vi "PNA-L_SET-CWFREQ.vi"(0 "Session In":refnum<visa-resource-name>="TCPIP0::K-Instr0000.local::hislip0::INSTR", 5 "error in":errorcluster {"code" format="%.0x"}, 6 "MODE":i32(ring) items=["Normal", "SMC"], 7 "FREQ":dbl=20.0 format="%#_6f", 8 "Timeout":u32=5000, 9 "Units":i64(ring)=1000000000 items=["GHz"=1000000000, "MHZ"=1000000], 10 "RO(T)":bool, 11 "CH":i32=3, 13 "Source":i32=1) -> (12 "freq":dbl=5.0, 14 "Session Out":refnum<visa-resource-name>="TCPIP0::K-Instr0000.local::hislip0::INSTR", 19 "error out":errorcluster {"code" format="%.0x"})   [LabVIEW 2018]
doc: "Applicable Models: All with Spectrum Analysis Options (S9x09xxA/B, S9x09xA/B)\n\n(Read-Write) Set and read the source CW frequency.\n \nParameters\n \n \n<ch>\n Any existing SA channel. If unspecified, value is set to 1.\n \n<port>\n Source port number of the VNA. If unspecified, value is set to 1. To make settings for ports that are not simple numbers, use the [src] argument.\n \n<num>\n CW frequency in Hz. Choose a value within the frequency range of the analyzer.\n \n[,src]\n String. (NOT case sensitive). Source port. Optional. Use SOUR:CAT? to return a list of valid port names.\n\nWhile this argument can be used to make settings for ALL ports, it is designed to access ports such as an external source, or one of the Source 2 outputs on the 2-port 2-source PNA-X model such as \"Port 1 Src2\". Otherwise, the <port> argument performs the same function. If both arguments are specified, [src] takes priority.\n \nExamples\n SENS:SA:SOUR:FREQ:CW 1e10\n\nsense2:sa:source:frequency:cw 1e9,\"Port 1 Src2\"\n \nQuery Syntax\n SENSe<ch>:SA:SOURce<port>:FREQuency:CW?\n \nReturn Type\n Numeric\n \nDefault\n Center frequency of the analyzer"
uses:
  lib functions/Agilent ENA Series.lvlib
  Agilent N5232A PNA-L/Labview Driver/Keysight PNA Series/Keysight PNA Series.lvlib
panel:
  out "concatenated string":string="sens3:sa:sour1:freq:cw?\nsens3:sa:sour1:freq:cw 5000000000.000000\n"
  # "Instrument Address"
  # "Meas Mode"
  # "Select Source"
  # "Conditions"
  # "Is Read Only (T)"
  # "Channel"
  # "Source"
  # "Inst Timeout(ms)"
  # "Set Freq"
  # "Freq"
  # "Read"
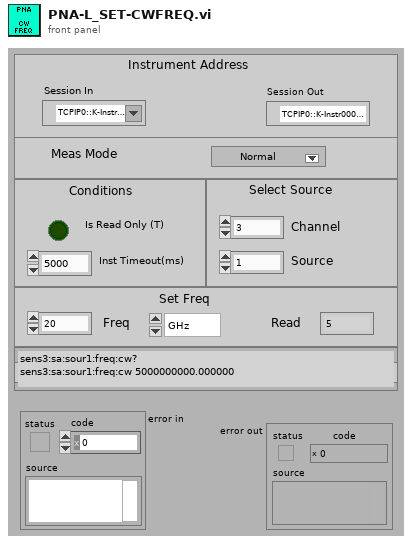
[diagram p1: front panel]
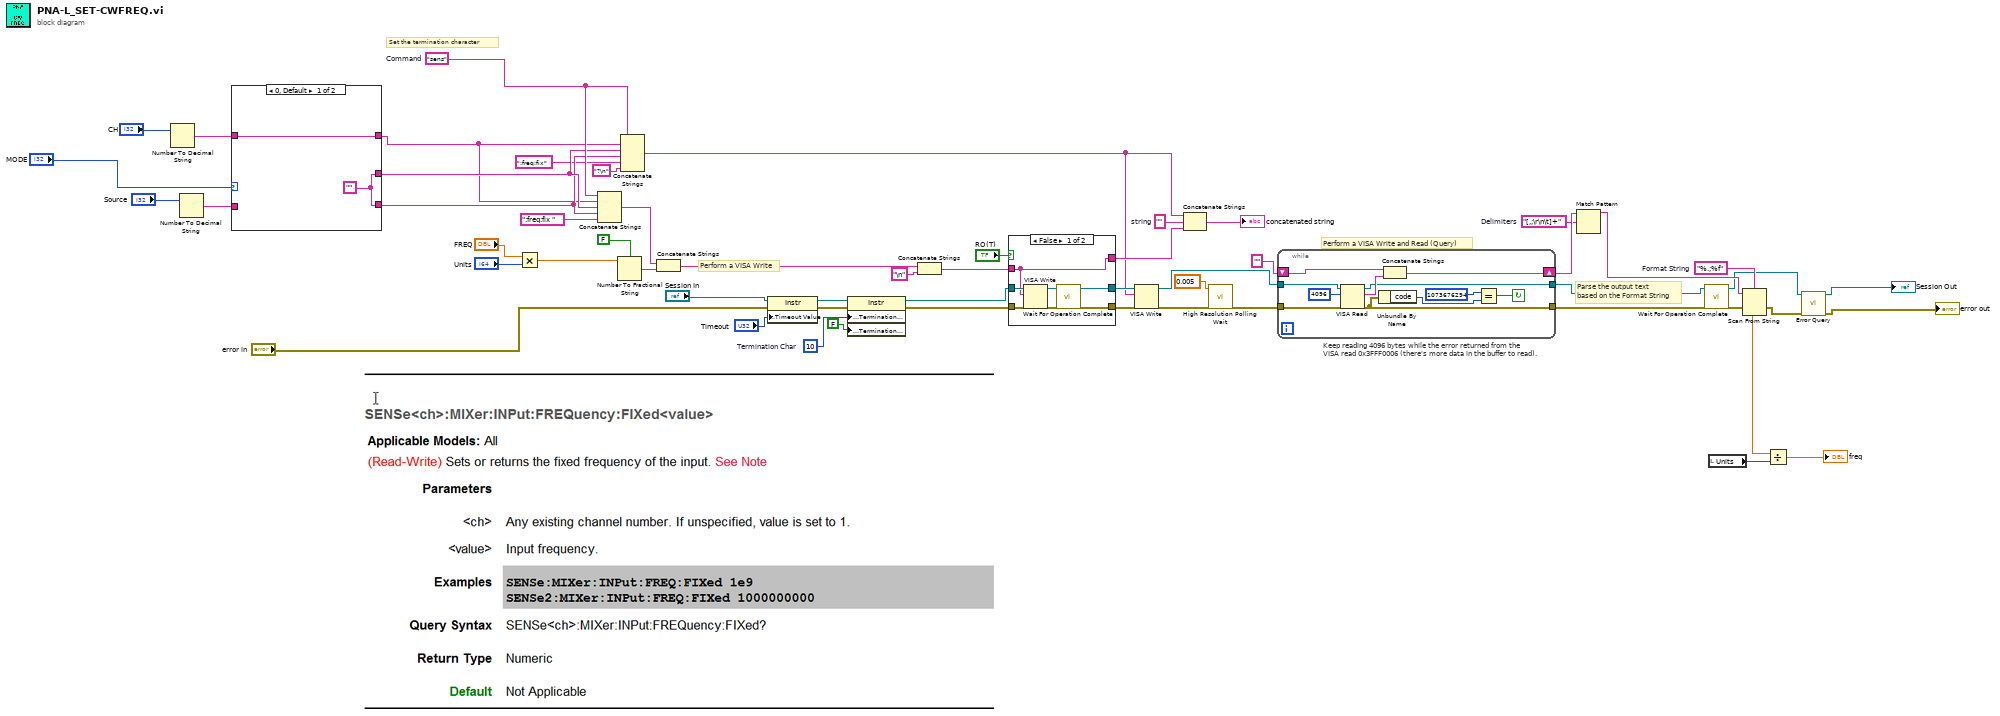
[diagram p0: block diagram]
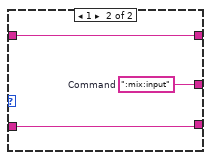
[diagram p2: hidden frame]
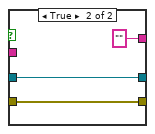
[diagram p3: hidden frame]
diagram:
  w34 = ""  # string
  w39 = "[,;\r\n\t]+"  # Delimiters
  w40 = "%.;%f"  # Format String
  w30 = "sens"  # Command
  w50 = u8 10  # Termination Char
  # "Parse the output text based on the Format String"
  # "Perform a VISA Write and Read (Query)"
  # "Keep reading 4096 bytes while the error returned from the\nVISA read 0x3FFF0006 (there's more data in the buffer to read)."
  # "Perform a VISA Write"
  # "Set the termination character"
  n1 = Number To Decimal String(number="CH") -> (decimal integer string=w6:string)  [unwired: 1 out]
  n2 = Number To Decimal String(number="Source") -> (decimal integer string=w7:string)  [unwired: 1 out]
  n3 = case shown="0, Default" "MODE" {
    tunnel: [w57 w61] -> w29
    tunnel: [w57 w60] -> w28
    tunnel: [w58 w59] -> w10
    tunnel: w7 -> [_ w60]
    tunnel: w6 -> [w58 w59]
    frame 0, Default {
      w57 = ""
    }
    frame 1 {
      w61 = ":mix:input"  # Command
    }
  }
  n4 = Multiply(x="FREQ", y="Units") -> (x*y=w25:dbl)
  n5 = Concatenate Strings(w30, w10, w29, w28, ":freq:fix " ("Command")) -> (w26:string)
  n6 = Number To Fractional String(use system decimal point (T)=FALSE, number=w25) -> (F-format string=w23:string)  [unwired: 2 in]
  n7 = Concatenate Strings(w30, w10, w29, w28, ":freq:fix" ("Command"), "?\n" ("Command")) -> (w18:string)
  n8 = Concatenate Strings(w26, w23) -> (w45:string)
  n9 = property class="Instr"(reference="Session In", error in="error in", "General Settings:Timeout Value"="Timeout") -> (reference out=w49:refnum<visa-resource-name>, error out=w52:errorcluster)
  n10 = property class="Instr"(reference=w49, error in=w52, "Message Based Settings:Termination Character"=w50, "Message Based Settings:Termination Character Enable"=FALSE ("enable")) -> (reference out=w38:refnum<visa-resource-name>, error out=w51:errorcluster)
  n11 = Concatenate Strings(w45, "\n" ("StaticText")) -> (w46:string)
  n12 = case shown="False" "RO(T)" {
    tunnel: w51 -> [w68 w70]
    tunnel: [w65 w70] -> w47
    tunnel: w46 -> [w66 _]
    tunnel: w38 -> [w67 w71]
    tunnel: [w62 w71] -> w37
    tunnel: [w66 ""] -> w19
    frame False {
      n13 = VISA Write(VISA resource name=w67, write buffer=w66, error in (no error)=w68) -> (VISA resource name out=w63:refnum<visa-resource-name>, error out=w64:errorcluster)  [unwired: 1 out]
      n14 = call "Wait For Operation Complete.vi"("error in (no error)"=w64, "VISA resource name"=w63) -> ("error out"=w65:errorcluster, "VISA resource name out"=w62:refnum<visa-resource-name>)  [unwired: 8 in]
    }
    frame True {
    }
  }
  n15 = VISA Write(VISA resource name=w37, write buffer=w18, error in (no error)=w47) -> (VISA resource name out=w15:refnum<visa-resource-name>, error out=w16:errorcluster)  [unwired: 1 out]
  n16 = Concatenate Strings(w18, w34, w19) -> (→"concatenated string":string)
  n17 = call <vilib>:"High Resolution Polling Wait.vi"("error in (no error)"=w16, "seconds to wait"=0.005) -> ("error out"=w17:errorcluster)  [unwired: 9 in]
  n18 = while {
    tunnel: w15 -> [w79]
    shift-right: [w73] -> w42
    shift-left: "" -> [w78]
    tunnel: w17 -> [w76]
    tunnel: [w75] -> w12
    tunnel: [w72] -> w13
    stop <- w74 continue-if-true
    n19 = VISA Read(VISA resource name=w79, byte count=u32 4096 ("byte count (0)"), error in (no error)=w76) -> (VISA resource name out=w72:refnum<visa-resource-name>, read buffer=w77:string, error out=w75:errorcluster)  [unwired: 1 out]
    n20 = Unbundle By Name(w75) -> ("code"=w81:i32)
    n21 = Concatenate Strings(w78, w77) -> (w73:string)
    n22 = Equal?(x=1073676294, y=w81) -> (x = y?=w74:bool)
  }
  n23 = Match Pattern(string=w42, regular expression=w39) -> (before substring=w41:string)  [unwired: 1 in, 3 out]
  n24 = call "Wait For Operation Complete.vi"("error in (no error)"=w12, "VISA resource name"=w13) -> ("error out"=w11:errorcluster, "VISA resource name out"=w1:refnum<visa-resource-name>)  [unwired: 8 in]
  n25 = local read "Units"() -> (w20:i64)
  n26 = Scan From String(format string=w40, input string=w41, error in=w11) -> (error out=w4:errorcluster, output 1=w32:dbl)  [unwired: 2 in, 2 out]
  n27 = Divide(x=w32, y=w20) -> (x/y=→"freq":dbl)
  n28 = call "Error Query.vi"("error in (no error)"=w4, "VISA resource name"=w1) -> ("error out"=→"error out":errorcluster, "VISA resource name out"=→"Session Out":refnum<visa-resource-name>)  [unwired: 6 in, 2 out]
